vi "var.vi"() -> ()   [LabVIEW 2020]
panel:
  out "B팀 점수":i8
  out "A팀 점수":i8
  out "전송 타임라인":string
  out "완성 문자":string
  # "글로벌 변수들"
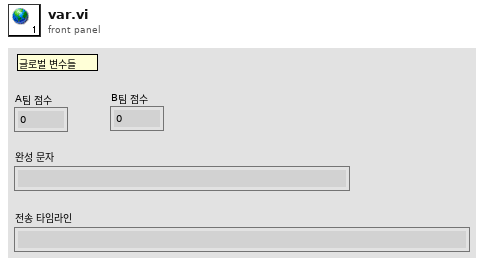
[diagram p1: front panel]
diagram:
